vi "DCIR@1C.vi"() -> ()   [LabVIEW 2020]
panel:
  out "DCIR@1C":dbl
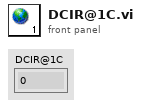
[diagram p1: front panel]
diagram:
